vi "low-pass filter.vi"(1 "smooth size":i32, 2 "Array 2":dbl[][](array[numeric])) -> (0 "Array":dbl[][](array[numeric]))   [LabVIEW 2009]
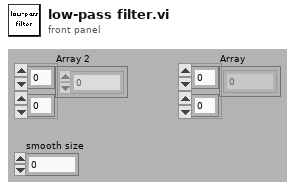
[diagram p1: front panel]
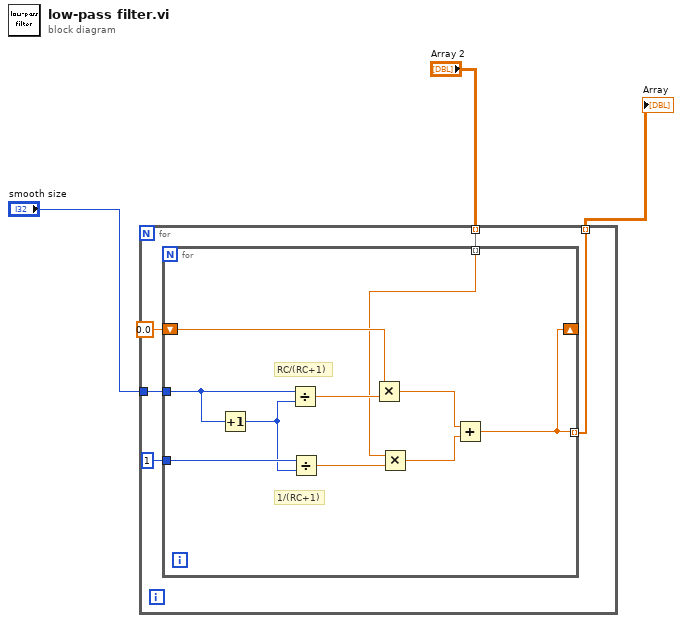
[diagram p0: block diagram]
diagram:
  n1 = for {
    tunnel: "smooth size" -> [w8]
    tunnel: "Array 2" -> [w6] mode=indexing
    tunnel: [w5] -> w3 mode=indexing
    n2 = for {
      shift-right: [w10] -> _
      shift-left: 0.0 -> [w18]
      tunnel: w8 -> [w15]
      tunnel: 1 ("smooth size") -> [w13]
      tunnel: [w10] -> w5 mode=indexing
      tunnel: w6 -> [w9] mode=indexing
      # "1/(RC+1)"
      # "RC/(RC+1)"
      n3 = Increment(x=w15) -> (x+1=w12:i32)
      n4 = Divide(x=w15, y=w12) -> (x/y=w14:dbl)
      n5 = Divide(x=w13, y=w12) -> (x/y=w11:dbl)
      n6 = Multiply(x=w18, y=w14) -> (x*y=w17:dbl)
      n7 = Multiply(x=w9, y=w11) -> (x*y=w16:dbl)
      n8 = Add(x=w17, y=w16) -> (x+y=w10:dbl)
    }
  }
  "Array" <- w3
